vi "5790A_config.vi"(4 "Input":enum16{"input 1", "input 2", "wide-band"}(ring), 5 "Digital filter mode":enum16{"off", "fast", "medium", "slow"}(ring), 6 "hi resolution":enum16{"off", "on"}(ring), 7 "Digital filter restart":enum16{"medium", "fine", "coarse"}(ring), 8 "error in":errorcluster, 11 "5790A":refnum<visa-resource-name>) -> (0 "error out":errorcluster, 3 "Session Out":refnum<visa-resource-name>)   [LabVIEW 2020]
doc: "Set value, frequency and function of Datron 4xxx series calibrators."
uses:
  <vilib>/Instr/_visa.llb/VISA GPIB Control REN Mode.ctl
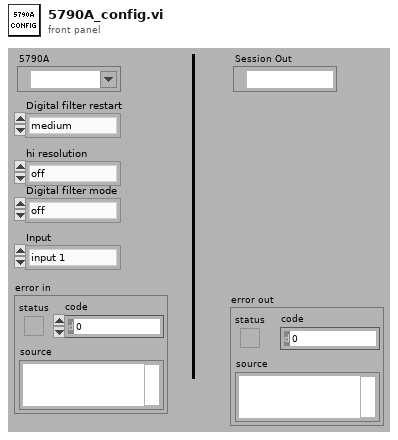
[diagram p1: front panel]
types:
  T1 = typedef "VISA GPIB Control REN Mode.ctl" = u16
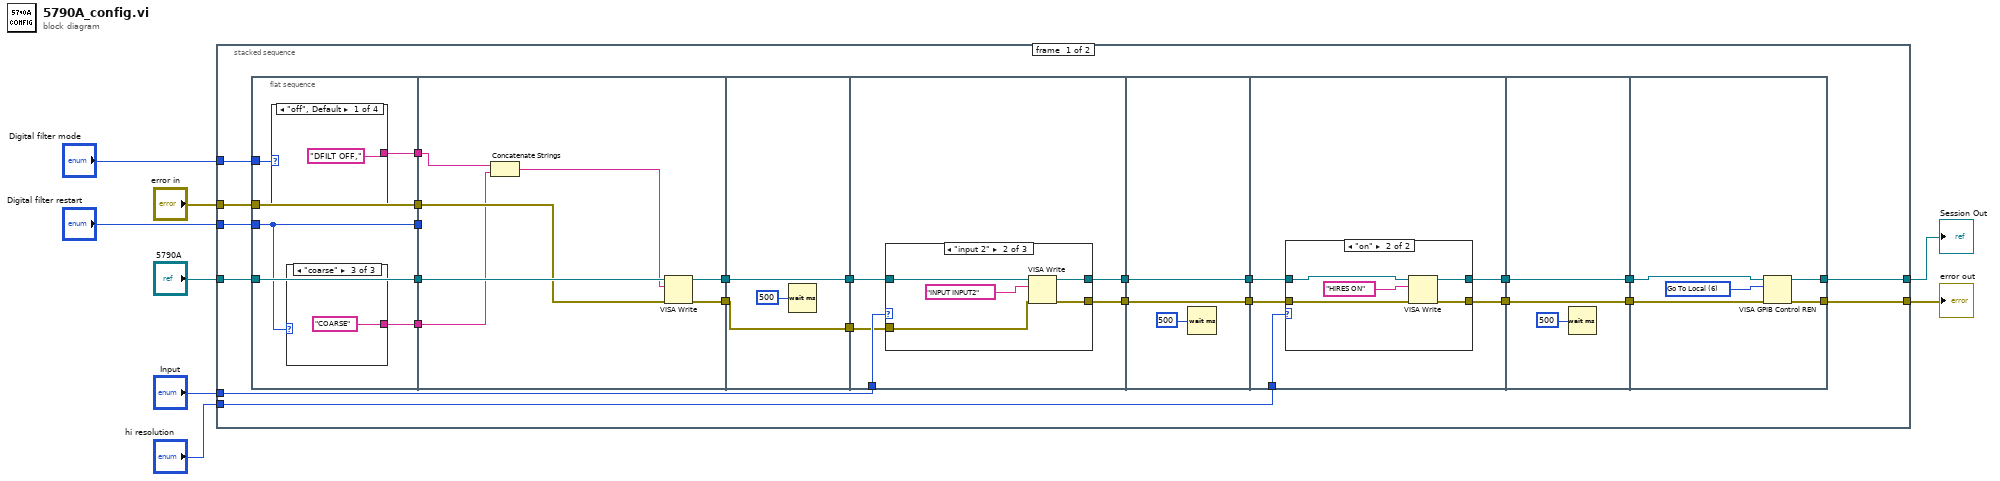
[diagram p0: block diagram]
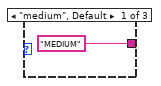
[diagram p2: hidden frame]
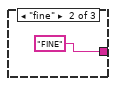
[diagram p3: hidden frame]
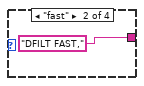
[diagram p4: hidden frame]
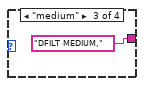
[diagram p5: hidden frame]
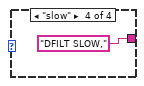
[diagram p6: hidden frame]
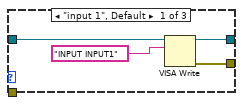
[diagram p7: hidden frame]
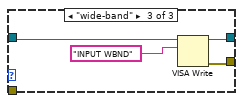
[diagram p8: hidden frame]
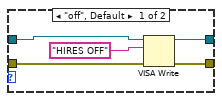
[diagram p9: hidden frame]
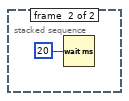
[diagram p10: hidden frame]
diagram:
  n1 = stacked-sequence {
    tunnel: "5790A" -> [w28 _]
    tunnel: "Digital filter restart" -> [w31 _]
    tunnel: [w33 _] -> w6
    tunnel: "error in" -> [w29 _]
    tunnel: [w32 _] -> w8
    tunnel: "Input" -> [w25 _]
    tunnel: "hi resolution" -> [w14 _]
    tunnel: "Digital filter mode" -> [w13 _]
    frame #0 {
      n2 = flat-sequence {
        tunnel: w28 -> [w38]
        tunnel: w29 -> [w37]
        tunnel: w31 -> [w35]
        tunnel: [w35] -> w23
        tunnel: [w37] -> w22
        tunnel: [w38] -> w21
        tunnel: w13 -> [w39]
        tunnel: [w36] -> w10
        tunnel: [w34] -> w9
        tunnel: [w52] -> w30
        tunnel: [w50] -> w11
        tunnel: w10 -> [w49]
        tunnel: w21 -> [w53]
        tunnel: w22 -> [w51]
        tunnel: w23 -> [_]
        tunnel: w9 -> [w48]
        tunnel: [w56] -> w24
        tunnel: w30 -> [w56]
        tunnel: [w54] -> w12
        tunnel: w11 -> [w54]
        tunnel: w24 -> [w58]
        tunnel: [w59] -> w27
        tunnel: [w60] -> w26
        tunnel: w25 -> [w61]
        tunnel: w12 -> [w57]
        tunnel: w27 -> [w77]
        tunnel: [w77] -> w20
        tunnel: w26 -> [w76]
        tunnel: [w76] -> w19
        tunnel: w20 -> [w78]
        tunnel: [w79] -> w18
        tunnel: w19 -> [w81]
        tunnel: [w80] -> w16
        tunnel: w14 -> [w82]
        tunnel: w18 -> [w95]
        tunnel: [w95] -> w17
        tunnel: w16 -> [w94]
        tunnel: [w94] -> w15
        tunnel: [w100] -> w33
        tunnel: [w99] -> w32
        tunnel: w17 -> [w97]
        tunnel: w15 -> [w96]
        frame #0 {
          n3 = case shown="\"off\", Default" w39 {
            tunnel: ["DFILT OFF," ("write buffer") "DFILT FAST," ("write buffer") "DFILT MEDIUM," ("write buffer") "DFILT SLOW," ("write buffer")] -> w36
            frame "off", Default {
            }
            frame "fast" {
            }
            frame "medium" {
            }
            frame "slow" {
            }
          }
          n4 = case shown="\"coarse\"" w35 {
            tunnel: ["MEDIUM" ("write buffer") "FINE" ("write buffer") "COARSE" ("write buffer")] -> w34
            frame "medium", Default {
            }
            frame "fine" {
            }
            frame "coarse" {
            }
          }
        }
        frame #1 {
          n5 = Concatenate Strings(w49, w48) -> (w47:string)
          n6 = VISA Write(VISA resource name=w53, write buffer=w47, error in (no error)=w51) -> (VISA resource name out=w52:refnum<visa-resource-name>, error out=w50:errorcluster)  [unwired: 1 out]
        }
        frame #2 {
          n7 = Wait (ms)(milliseconds to wait=u32 500) -> ()  [unwired: 1 out]
        }
        frame #3 {
          n8 = case shown="\"input 2\"" w61 {
            tunnel: [w64 w70 w73] -> w60
            tunnel: [w63 w69 w72] -> w59
            tunnel: w58 -> [w65 w68 w71]
            tunnel: w57 -> [_ w66 _]
            frame "input 1", Default {
              n9 = VISA Write(VISA resource name=w65, write buffer="INPUT INPUT1") -> (VISA resource name out=w63:refnum<visa-resource-name>, error out=w64:errorcluster)  [unwired: 1 in, 1 out]
            }
            frame "input 2" {
              n10 = VISA Write(VISA resource name=w68, write buffer="INPUT INPUT2", error in (no error)=w66) -> (VISA resource name out=w69:refnum<visa-resource-name>, error out=w70:errorcluster)  [unwired: 1 out]
            }
            frame "wide-band" {
              n11 = VISA Write(VISA resource name=w71, write buffer="INPUT WBND") -> (VISA resource name out=w72:refnum<visa-resource-name>, error out=w73:errorcluster)  [unwired: 1 in, 1 out]
            }
          }
        }
        frame #4 {
          n12 = Wait (ms)(milliseconds to wait=u32 500) -> ()  [unwired: 1 out]
        }
        frame #5 {
          n13 = case shown="\"on\"" w82 {
            tunnel: w81 -> [w86 w92]
            tunnel: [w85 w91] -> w80
            tunnel: [w84 w90] -> w79
            tunnel: w78 -> [w87 w89]
            frame "off", Default {
              n14 = VISA Write(VISA resource name=w87, write buffer="HIRES OFF", error in (no error)=w86) -> (VISA resource name out=w84:refnum<visa-resource-name>, error out=w85:errorcluster)  [unwired: 1 out]
            }
            frame "on" {
              n15 = VISA Write(VISA resource name=w89, write buffer="HIRES ON", error in (no error)=w92) -> (VISA resource name out=w90:refnum<visa-resource-name>, error out=w91:errorcluster)  [unwired: 1 out]
            }
          }
        }
        frame #6 {
          n16 = Wait (ms)(milliseconds to wait=u32 500) -> ()  [unwired: 1 out]
        }
        frame #7 {
          w98 = T1 6 items=["Deassert REN", "Assert REN", "Go To Local; Deassert REN ", "Assert REN; Address Device", "Local Lockout (Addressed Devices)", "Local Lockout (This Device)", "Go To Local"] ("Mode")
          n17 = VISA GPIB Control REN(8:w96, 10:w98, 11:w97) -> (0:w100:errorcluster, 3:w99:refnum<visa-resource-name>)
        }
      }
    }
    frame #1 {
      n18 = Wait (ms)(milliseconds to wait=u32 20 ("millisecond multiple")) -> ()  [unwired: 1 out]
    }
  }
  "Session Out" <- w8
  "error out" <- w6
